vi "Flyout Window.vi"(10 "Boolean in":refnum<vi>) -> (1 "Cancelled?":bool=TRUE, 2 "Sensor Out":refnum<class "Sensor.lvclass">, 4 "AutoStart?":bool=TRUE)   [LabVIEW 2012, in "Win8uiDemo.lvlib" / "Flyout.lvclass"]
uses:
  Flyout.lvclass
  <vilib>/ActorFramework/Message Enqueuer/Message Enqueuer.lvclass
  Sensor Definition/Sensor.lvclass
  Vertical Alignment.ctl
  Horizontal Alignment.ctl
  Sensor Definition/SensorInfo.lvclass
  TimerSensor/TimerSensor.lvclass
  TimerSensor/TimerSensorConfig.lvclass
  Sensor Definition/SensorInfo.lvclass/SensorInfo.ctl
  Sensor Definition/Sensor.lvclass/Sensor.ctl
  Sensor Definition/SensorInfo/Write Name.vi
  Sensor Definition/Write Description.vi
  Sensor Definition/SensorInfo/Write Config.vi
  Sensor Definition/Sensor/Write SensorInfo.vi
panel:
  in  "Sensor":u16(ring) items=["Sensor", "Timer"]
  in  "Description":string="Name"
  out "Title":string="Settings"
  in  "Name":string="Name"
  in  "Reciever":refnum<class "Message Enqueuer.lvclass">
  in  "Button":bool
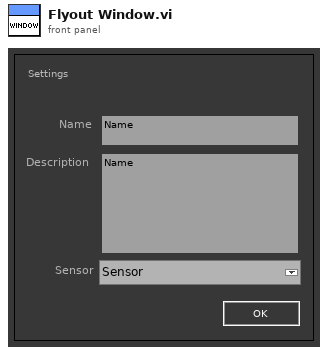
[diagram p1: front panel]
types:
  T1 = enum32{"Invalid", "Standard", "Closed", "Hidden", "Minimized", "Maximized"}
  T2 = typedef "Win8uiDemo.lvlib/Flyout.lvclass/Horizontal Alignment.ctl" = enum16{"Centered", "Left", "Right"}
  T3 = typedef "Win8uiDemo.lvlib/Flyout.lvclass/Vertical Alignment.ctl" = enum16{"Centered", "Above", "Below"}
  T4 = typedef "LVPointTypeDef.ctl" = cluster{"Horizontal":i16, "Vertical":i16}
  T5 = typedef "LVRectTypeDef.ctl" = cluster{"Left":i16, "Top":i16, "Right":i16, "Bottom":i16}
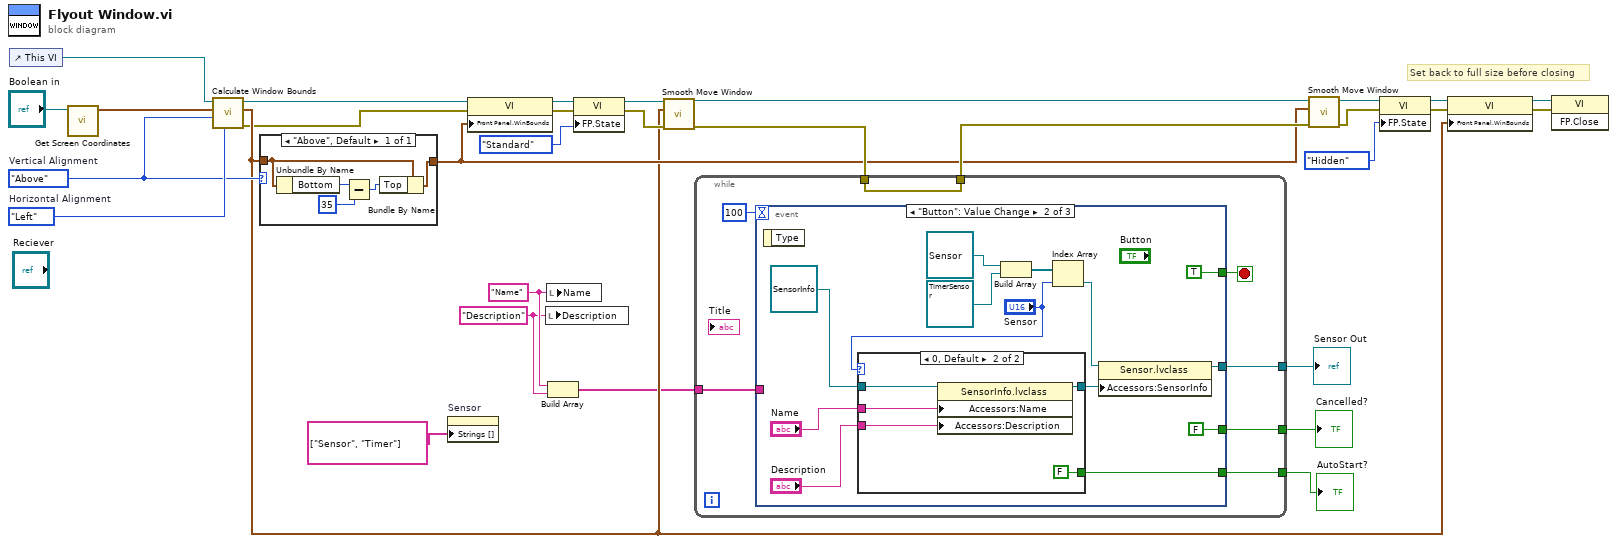
[diagram p0: block diagram]
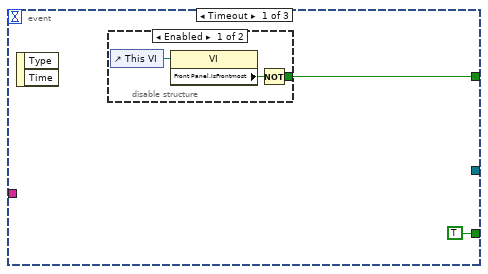
[diagram p2: hidden frame]
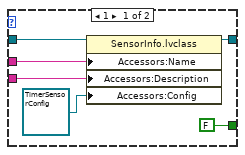
[diagram p4: hidden frame]
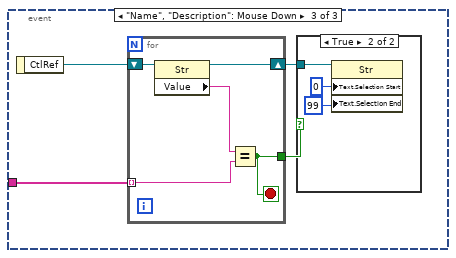
[diagram p5: hidden frame]
diagram:
  w6 = "Description" ("Description")
  w7 = "Name" ("Name")
  w30 = Horizontal_Alignment."Left"  # Horizontal Alignment
  w23 = Vertical_Alignment."Above"  # Vertical Alignment
  # "Set back to full size before closing"
  n1 = control-ref of="This VI"() -> (w29:refnum<vi>)
  n2 = call "Get Screen Coordinates.vi"("Boolean in"="Boolean in") -> ("ScreenCoords"=w11:T4)  [unwired: 9 in, 1 out]
  n3 = call "Calculate Window Bounds.vi"("Horizontal Alignment"=w30, "Vertical Alignment"=w23, "Position (Screen)"=w11, "VI in"=w29) -> ("error out"=w3:errorcluster, "Front Panel Window:Window Bounds"=w14:T5, "VI out"=w28:refnum<vi>)  [unwired: 5 in]
  n4 = case shown="\"Above\", Default" w23 {
    tunnel: w14 -> [w33]
    tunnel: [w32] -> w20
    frame "Above", Default {
      n5 = Unbundle By Name(w33) -> ("Bottom"=w36:i16)
      n6 = Subtract(x=w36, y=i16 35) -> (x-y=w34:i16)
      n7 = Bundle By Name(cluster=w33, "Top"=w34) -> (w32:T5)
    }
  }
  n8 = property on="Sensor" class="Ring (strict)"("Strings []"=string[] ["Sensor", "Timer"]) -> ()  [unwired: 2 in, 2 out]
  n9 = property class="VI"(reference=w28, error in=w3, "Front Panel.WinBounds"=w20) -> (reference out=w27:refnum<vi>, error out=w26:errorcluster)
  n10 = local write "Description"(w6) -> ()
  n11 = local write "Name"(w7) -> ()
  n12 = Build Array(w7, w6) -> (w5:string[])
  n13 = property class="VI"(reference=w27, error in=w26, "FP.State"=T1."Standard" ("Front Panel Window:State")) -> (reference out=w24:refnum<vi>, error out=w19:errorcluster)
  n14 = call "Smooth Move Window.vi"("error in (no error)"=w19, "Front Panel Window:Window Bounds"=w14, "VI in"=w24) -> ("error out"=w31:errorcluster, "VI out"=w21:refnum<vi>)  [unwired: 7 in]
  n15 = while {
    tunnel: w31 -> [w41]
    tunnel: [w41] -> w22
    tunnel: [w40] -> w9
    tunnel: [w39] -> w8
    tunnel: w5 -> [w38]
    tunnel: [w37] -> w1
    stop <- w42 stop-if-true
    n16 = event shown="[1] \"Button\": Value Change" {
      selector: _ -> [_ _ _]
      dyn-events: _ -> [_ _ _]
      timeout: 100 -> [_ _ _]
      tunnel: [w45 TRUE _] -> w42
      tunnel: [_ w56 _] -> w40
      tunnel: [TRUE FALSE _] -> w39
      tunnel: w38 -> [_ _ w75]
      tunnel: [_ w49 _] -> w37
      event Timeout {
        n17 = event-data() -> ()  [unwired: 1 in, 2 out]
        n18 = disable-structure shown="Enabled" {
          disable-tunnel: [w46 _] -> w45
          frame Enabled {
            n19 = control-ref of="This VI"() -> (w47:refnum<vi>)
            n20 = property class="VI"(reference=w47) -> ("Front Panel.IsFrontmost"=w48:bool)  [unwired: 1 in, 2 out]
            n21 = Not(x=w48) -> (.not. x?=w46:bool)
          }
          frame Disabled {
          }
        }
      }
      event "Button": Value Change {
        n22 = event-data() -> ()  [unwired: 1 in, 1 out]
        n23 = case shown="0, Default" "Sensor" {
          tunnel: refnum<class "SensorInfo.lvclass"> refnum ("SensorInfo") -> [w67 w72]
          tunnel: [w66 w71] -> w59
          tunnel: "Name" -> [w65 w70]
          tunnel: "Description" -> [w64 w69]
          tunnel: [FALSE FALSE] -> w49
          frame 1 {
            n24 = property class="SensorInfo.lvclass"(reference=w67, "Accessors:Name"=w65, "Accessors:Description"=w64, "Accessors:Config"=refnum<class "TimerSensorConfig.lvclass"> refnum ("TimerSensor.lvlib:TimerSensorConfig.lvclass")) -> (reference out=w66:refnum<class "SensorInfo.lvclass">)  [unwired: 1 in, 1 out]
          }
          frame 0, Default {
            n25 = property class="SensorInfo.lvclass"(reference=w72, "Accessors:Name"=w70, "Accessors:Description"=w69) -> (reference out=w71:refnum<class "SensorInfo.lvclass">)  [unwired: 1 in, 1 out]
          }
        }
        n26 = Build Array(refnum<class "Sensor.lvclass"> refnum ("Sensor Definition.lvlib:Sensor.lvclass"), refnum<class "TimerSensor.lvclass"> refnum ("TimerSensor.lvlib:TimerSensor.lvclass")) -> (w52:refnum<class "Sensor.lvclass">[])
        n27 = Index Array(array=w52, index="Sensor") -> (element=w51:refnum<class "Sensor.lvclass">)
        n28 = property class="Sensor.lvclass"(reference=w51, "Accessors:SensorInfo"=w59) -> (reference out=w56:refnum<class "Sensor.lvclass">)  [unwired: 1 in, 1 out]
      }
      event "Name", "Description": Mouse Down {
        n29 = event-data() -> ("CtlRef"=w76:refnum<vi>)  [unwired: 1 in]
        n30 = for {
          tunnel: w75 -> [w83] mode=indexing
          tunnel: [w80] -> w73
          shift-right: [w81] -> w74
          shift-left: w76 -> [w84]
          stop <- w80 stop-if-true
          n31 = property class="Str"(reference=w84) -> (reference out=w81:refnum<vi>, "Value"=w82:string)  [unwired: 1 in, 1 out]
          n32 = Equal?(x=w82, y=w83) -> (x = y?=w80:bool)
        }
        n33 = case shown="True" w73 {
          tunnel: w74 -> [_ w79]
          frame False {
          }
          frame True {
            n34 = property class="Str"(reference=w79, "Text.Selection Start"=u32 0 ("Text.Selection:Start"), "Text.Selection End"=u32 99 ("Text.Selection:Start")) -> ()  [unwired: 1 in, 2 out]
          }
        }
      }
    }
  }
  "Sensor Out" <- w9
  "Cancelled?" <- w8
  "AutoStart?" <- w1
  n35 = call "Smooth Move Window.vi"("error in (no error)"=w22, "Front Panel Window:Window Bounds"=w20, "VI in"=w21) -> ("error out"=w4:errorcluster, "VI out"=w18:refnum<vi>)  [unwired: 7 in]
  n36 = property class="VI"(reference=w18, error in=w4, "FP.State"=T1."Hidden" ("Front Panel Window:State")) -> (reference out=w16:refnum<vi>, error out=w15:errorcluster)
  n37 = property class="VI"(reference=w16, error in=w15, "Front Panel.WinBounds"=w14) -> (reference out=w13:refnum<vi>, error out=w12:errorcluster)
  n38 = invoke class="VI" method="FP.Close"(reference=w13, error in=w12) -> ()  [unwired: 1 in, 3 out]
